vi "LOC subReadWriteVIStringINIKeys.vi"(4 "DebugLOC":bool, 5 "Mode":enum16{"Read", "Write"}(ring), 6 "error in (no error)":errorcluster, 7 "ConfigFileRefnum":T1, 8 "VIName":string, 9 "ControlRefnums":refnum<vi>[](array[refnum])) -> (0 "error out":errorcluster)   [LabVIEW 2020, in "Localization_Tools.lvlib"]
uses:
  Localization_Tools.lvlib
  <vilib>/Utility/config.llb/Config Data RefNum.ctl
  <vilib>/Utility/config.llb/NI_LVConfig.lvlib
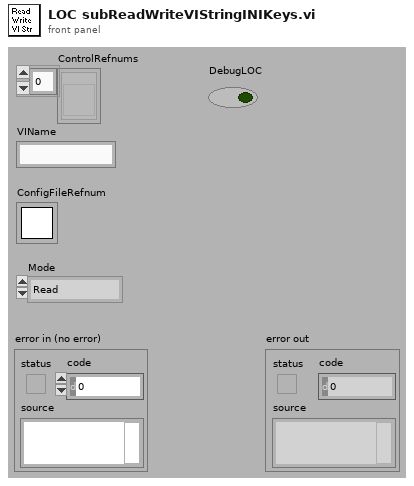
[diagram p1: front panel]
types:
  T1 = typedef "NI_LVConfig.lvlib/Config Data RefNum.ctl" = refnum<k1>
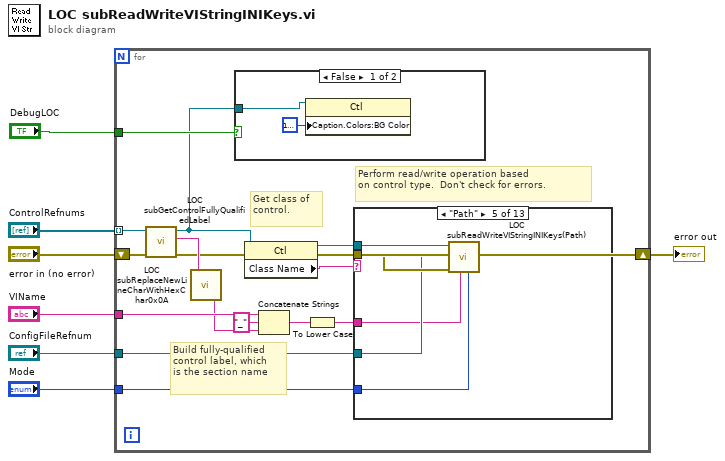
[diagram p0: block diagram]
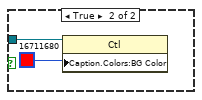
[diagram p2: hidden frame]
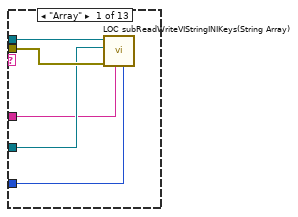
[diagram p3: hidden frame]
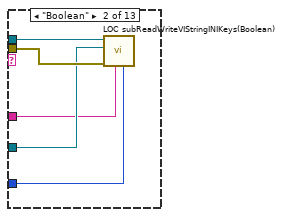
[diagram p4: hidden frame]
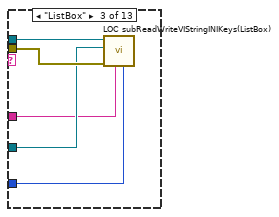
[diagram p5: hidden frame]
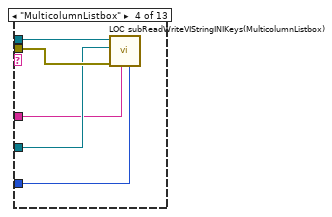
[diagram p6: hidden frame]
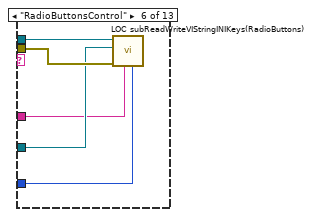
[diagram p7: hidden frame]
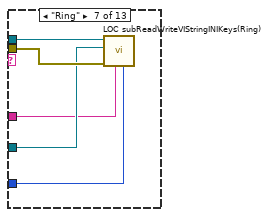
[diagram p8: hidden frame]
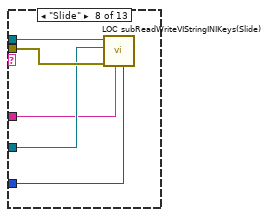
[diagram p9: hidden frame]
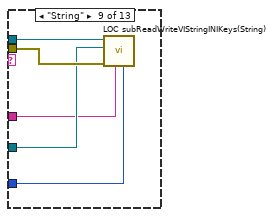
[diagram p10: hidden frame]
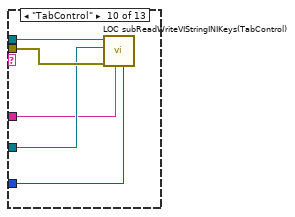
[diagram p11: hidden frame]
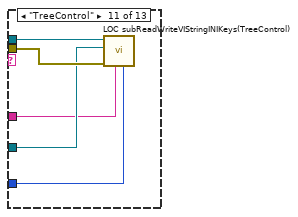
[diagram p12: hidden frame]
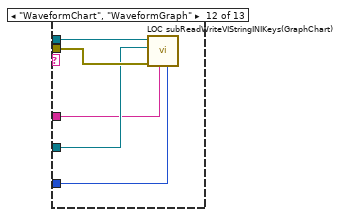
[diagram p13: hidden frame]
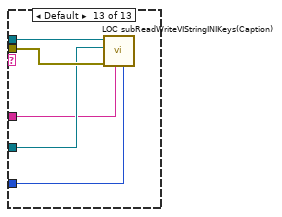
[diagram p14: hidden frame]
diagram:
  n1 = for {
    tunnel: "ControlRefnums" -> [w21] mode=indexing
    tunnel: "VIName" -> [w23]
    tunnel: "ConfigFileRefnum" -> [w14]
    tunnel: "Mode" -> [w15]
    shift-right: [w12] -> w2
    shift-left: "error in (no error)" -> [w13]
    tunnel: "DebugLOC" -> [w10]
    # "Perform read/write operation based\non control type.  Don't check for errors."
    # "Build fully-qualified\ncontrol label, which\nis the section name"
    # "Get class of\ncontrol."
    n2 = call "LOC subGetControlFullyQualifiedLabel.vi"("error in (no error)"=w13, "reference"=w21) -> ("error out"=w18:errorcluster, "Fully Qualified Label"=w20:string, "dup reference"=w9:refnum<vi>)  [unwired: 3 in]
    n3 = call "LOC subReplaceNewLineCharWithHexChar0x0A.vi"("InputString"=w20) -> ("OutputString"=w19:string)
    n4 = case shown="False" w10 {
      tunnel: w9 -> [w25 w27]
      frame False {
        n5 = property class="Ctl"(reference=w25, "Caption.Colors:BG Color"=u32 16777216) -> ()  [unwired: 1 in, 2 out]
      }
      frame True {
        n6 = property class="Ctl"(reference=w27, "Caption.Colors:BG Color"=u32 16711680) -> ()  [unwired: 1 in, 2 out]
      }
    }
    n7 = property class="Ctl"(reference=w9, error in=w18) -> (reference out=w16:refnum<vi>, error out=w12:errorcluster, "Class Name"=w17:string)
    n8 = Concatenate Strings(w23, "_" ("string"), w19) -> (w11:string)
    n9 = To Lower Case(string=w11) -> (all lower case string=w8:string)
    n10 = case shown="\"Path\"" w17 {
      tunnel: w8 -> [w28 w33 w38 w43 w48 w53 w58 w63 w68 w73 w78 w83 w88]
      tunnel: w16 -> [w32 w37 w42 w47 w52 w57 w62 w67 w72 w77 w82 w87 w92]
      tunnel: w12 -> [w31 w36 w41 w46 w51 w56 w61 w66 w71 w76 w81 w86 w91]
      tunnel: w15 -> [w29 w34 w39 w44 w49 w54 w59 w64 w69 w74 w79 w84 w89]
      tunnel: w14 -> [w30 w35 w40 w45 w50 w55 w60 w65 w70 w75 w80 w85 w90]
      frame "Array" {
        n11 = call "LOC subReadWriteVIStringINIKeys(String Array).vi"("Mode"=w29, "Section"=w28, "error in (no error)"=w31, "ConfigFileRefnum"=w30, "ControlRefnum"=w32) -> ()  [unwired: 4 in, 1 out]
      }
      frame "Boolean" {
        n12 = call "LOC subReadWriteVIStringINIKeys(Boolean).vi"("Mode"=w34, "Section"=w33, "error in (no error)"=w36, "ConfigFileRefnum"=w35, "ControlRefnum"=w37) -> ()  [unwired: 4 in, 1 out]
      }
      frame "ListBox" {
        n13 = call "LOC subReadWriteVIStringINIKeys(ListBox).vi"("Mode"=w39, "Section"=w38, "error in (no error)"=w41, "ConfigFileRefnum"=w40, "ControlRefnum"=w42) -> ()  [unwired: 4 in, 1 out]
      }
      frame "MulticolumnListbox" {
        n14 = call "LOC subReadWriteVIStringINIKeys(MulticolumnListbox).vi"("Mode"=w44, "Section"=w43, "error in (no error)"=w46, "ConfigFileRefnum"=w45, "ControlRefnum"=w47) -> ()  [unwired: 4 in, 1 out]
      }
      frame "Path" {
        n15 = call "LOC subReadWriteVIStringINIKeys(Path).vi"("Mode"=w49, "Section"=w48, "error in (no error)"=w51, "ConfigFileRefnum"=w50, "ControlRefnum"=w52) -> ()  [unwired: 4 in, 1 out]
      }
      frame "RadioButtonsControl" {
        n16 = call "LOC subReadWriteVIStringINIKeys(RadioButtons).vi"("Mode"=w54, "Section"=w53, "error in (no error)"=w56, "ConfigFileRefnum"=w55, "ControlRefnum"=w57) -> ()  [unwired: 4 in, 1 out]
      }
      frame "Ring" {
        n17 = call "LOC subReadWriteVIStringINIKeys(Ring).vi"("Mode"=w59, "Section"=w58, "error in (no error)"=w61, "ConfigFileRefnum"=w60, "ControlRefnum"=w62) -> ()  [unwired: 4 in, 1 out]
      }
      frame "Slide" {
        n18 = call "LOC subReadWriteVIStringINIKeys(Slide).vi"("Mode"=w64, "Section"=w63, "error in (no error)"=w66, "ConfigFileRefnum"=w65, "ControlRefnum"=w67) -> ()  [unwired: 4 in, 1 out]
      }
      frame "String" {
        n19 = call "LOC subReadWriteVIStringINIKeys(String).vi"("Mode"=w69, "Section"=w68, "error in (no error)"=w71, "ConfigFileRefnum"=w70, "ControlRefnum"=w72) -> ()  [unwired: 4 in, 1 out]
      }
      frame "TabControl" {
        n20 = call "LOC subReadWriteVIStringINIKeys(TabControl).vi"("Mode"=w74, "Section"=w73, "error in (no error)"=w76, "ConfigFileRefnum"=w75, "ControlRefnum"=w77) -> ()  [unwired: 4 in, 1 out]
      }
      frame "TreeControl" {
        n21 = call "LOC subReadWriteVIStringINIKeys(TreeControl).vi"("Mode"=w79, "Section"=w78, "error in (no error)"=w81, "ConfigFileRefnum"=w80, "ControlRefnum"=w82) -> ()  [unwired: 4 in, 1 out]
      }
      frame "WaveformChart", "WaveformGraph" {
        n22 = call "LOC subReadWriteVIStringINIKeys(GraphChart).vi"("Mode"=w84, "Section"=w83, "error in (no error)"=w86, "ConfigFileRefnum"=w85, "ControlRefnum"=w87) -> ()  [unwired: 4 in, 1 out]
      }
      frame Default {
        n23 = call "LOC subReadWriteVIStringINIKeys(Caption).vi"("Mode"=w89, "Section"=w88, "error in (no error)"=w91, "ConfigFileRefnum"=w90, "ControlRefnum"=w92) -> ()  [unwired: 3 in, 2 out]
      }
    }
  }
  "error out" <- w2
